vi "Simulation24Q1.vi"() -> ()   [LabVIEW 2024]
panel:
  out "out":dbl
  in  "in":dbl
  in  "function name":string
  in  "module path":path
  in  "Python path":path
  in  "Python version":string
  out "A2P":bool(c317)
  out "Actuator Valve 2":bool
  out "A1P":bool(c317)
  in  "Actuator Valve 1":bool
  out "Multi-Segment Pipe 5":bool(c317)
  out "A2_pipe":bool(c317)
  out "A1_pipe":bool(c317)
  out "Multi-Segment Pipe 10":bool(c317)
  out "Multi-Segment Pipe 9":bool(c317)
  in  "stop":bool
  in  "Oil Pump":bool
  out "S2":bool
  out "S1":bool
  out "Tank 2":dbl(slide) scale=0.0..100.0
  out "Multi-Segment Pipe 7":bool(c317)
  out "Multi-Segment Pipe 6":bool(c317)
  out "Multi-Segment Pipe 4":bool(c317)
  out "Multi-Segment Pipe 3":bool(c317)
  out "Multi-Segment Pipe 2":bool(c317)
  out "Tank 1":dbl(slide) scale=0.0..100.0
  # "Level Sensor"
  # "Oil Source"
  # "Level Sensor"
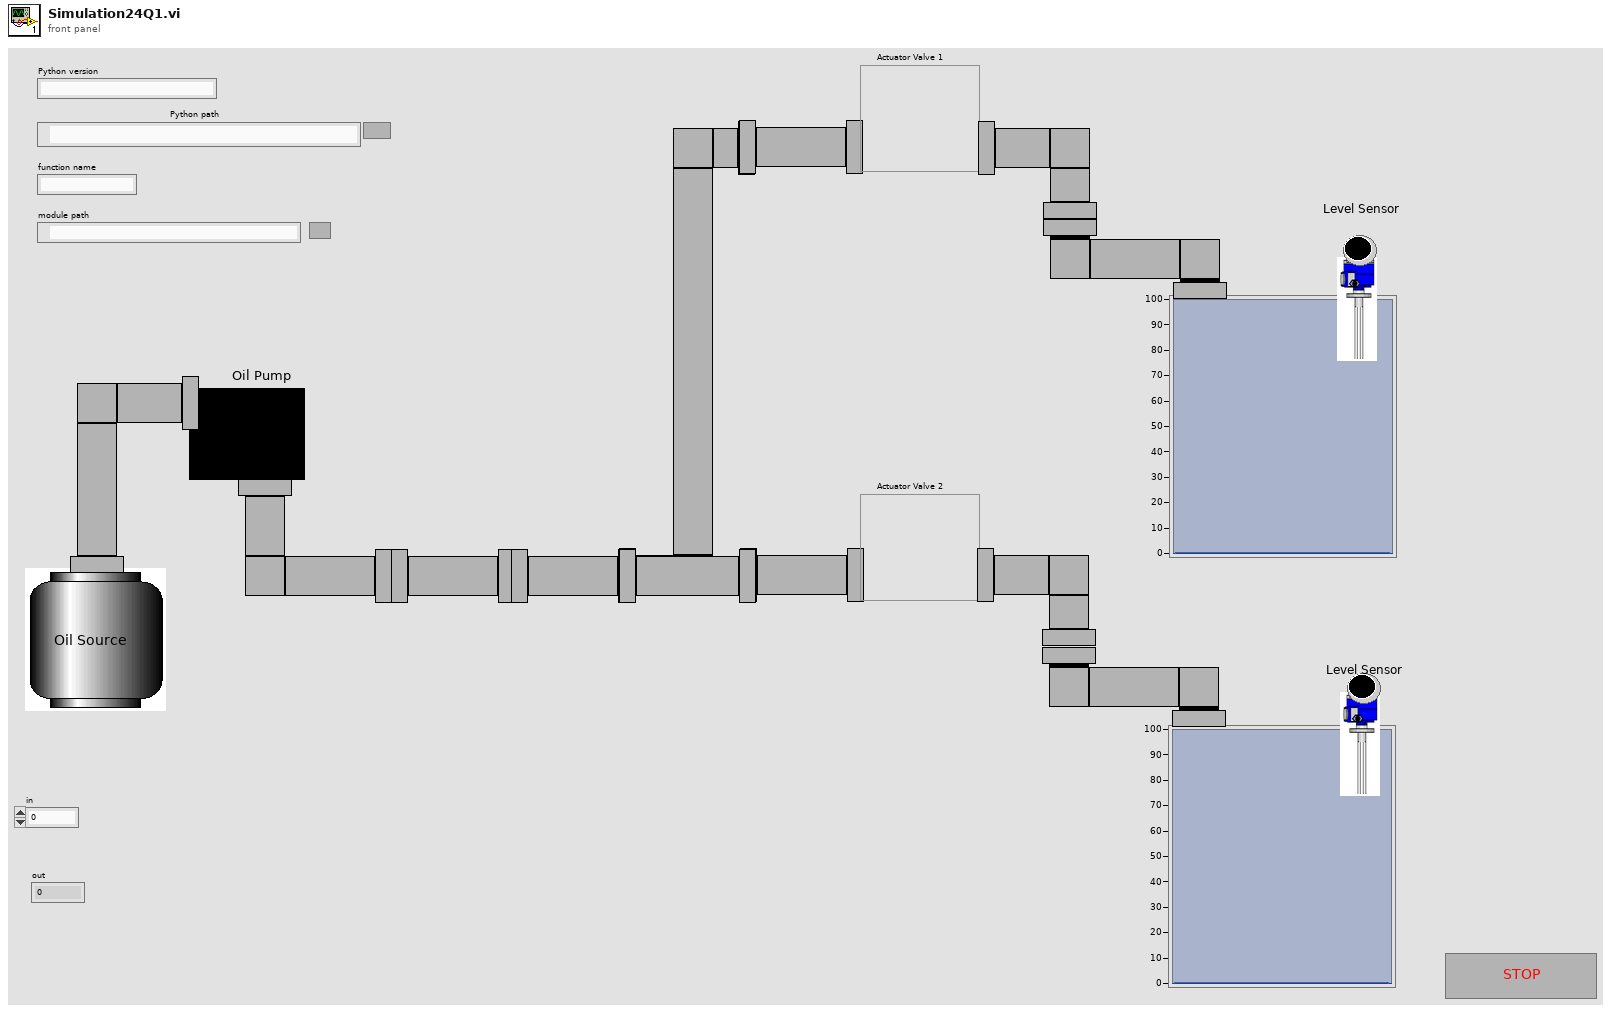
[diagram p1: front panel]
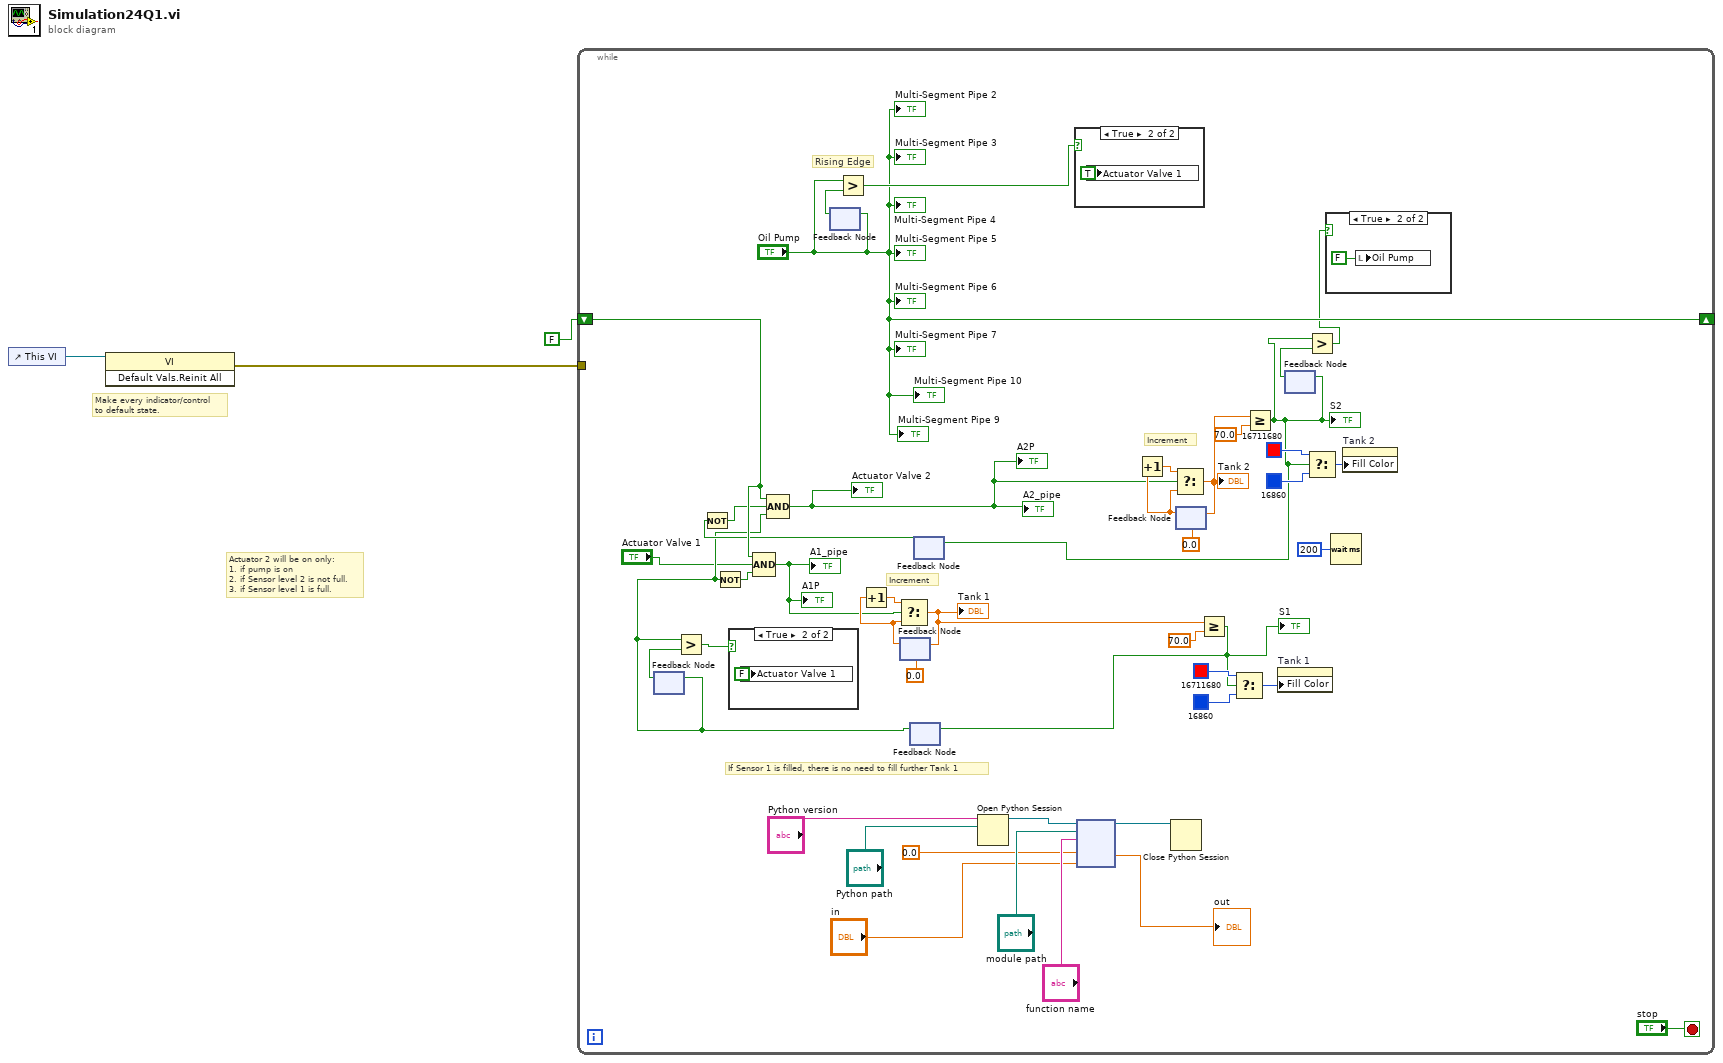
[diagram p0: block diagram]
diagram:
  # "Actuator 2 will be on only:\n1. if pump is on\n2. if Sensor level 2 is not full.\n3. if Sensor level 1 is full."
  # "Make every indicator/control\nto default state."
  n1 = control-ref of="This VI"() -> (w2:refnum<vi>)
  n2 = invoke class="VI" method="Default Vals.Reinit All"(reference=w2) -> (error out=w1:errorcluster)  [unwired: 2 in, 2 out]
  n3 = while {
    shift-right: ["Oil Pump"] -> _
    shift-left: FALSE -> [w46]
    tunnel: w1 -> [_]
    stop <- "stop" stop-if-true
    # "Increment"
    # "Increment"
    # "If Sensor 1 is filled, there is no need to fill further Tank 1"
    # "Rising Edge"
    n4 = feedback #1() -> (w28:bool)  [unwired: 1 in]
    n5 = feedback #2() -> (w22:bool)  [unwired: 1 in]
    n6 = feedback-in #2("Oil Pump") -> ()
    n7 = Greater?(x="Oil Pump", y=w22) -> (0:w21:bool)
    n8 = feedback #3(0.0) -> (w41:dbl)
    n9 = Increment(x=w41) -> (x+1=w40:dbl)
    n10 = feedback #4() -> (w23:bool)  [unwired: 1 in]
    n11 = feedback-in #1(w23) -> ()
    n12 = Greater?(x=w23, y=w28) -> (0:w27:bool)
    n13 = Not(x=w23) -> (.not. x?=w26:bool)
    n14 = case shown="True" w27 {
      frame False {
      }
      frame True {
        n15 = local write "Actuator Valve 1"(FALSE ("Actuator 1")) -> ()
      }
    }
    n16 = Compound Arithmetic op=AND(w46, "Actuator Valve 1", w26) -> (w16:bool)
    "A1_pipe" <- w16
    "A1P" <- w16
    n17 = Select(t=w40, s=w16, f=w41) -> (s? t:f=w7:dbl)
    "Tank 1" <- w7
    n18 = feedback-in #3(w7) -> ()
    n19 = feedback #5() -> (w25:bool)  [unwired: 1 in]
    n20 = Not(x=w25) -> (.not. x?=w24:bool)
    n21 = Compound Arithmetic op=AND(w46, w24, w23) -> (w14:bool)
    "A2_pipe" <- w14
    "Actuator Valve 2" <- w14
    "A2P" <- w14
    n22 = Open Python Session(python version="Python version", python path="Python path") -> (session out=w11:refnum<k35>)  [unwired: 1 in, 1 out]
    n23 = case shown="True" w21 {
      frame False {
      }
      frame True {
        n24 = local write "Actuator Valve 1"(TRUE ("Actuator 1")) -> ()
      }
    }
    n25 = node(w11, "module path", "function name", 0.0, "in") -> (w8:refnum<k35>, →"out":dbl)  [unwired: 2 in, 3 out]
    n26 = Close Python Session(session in=w8) -> ()  [unwired: 1 in, 1 out]
    n27 = feedback #6(0.0) -> (w42:dbl)
    n28 = Increment(x=w42) -> (x+1=w43:dbl)
    n29 = Select(t=w43, s=w14, f=w42) -> (s? t:f=w38:dbl)
    "Tank 2" <- w38
    n30 = feedback-in #6(w38) -> ()
    n31 = Greater Or Equal?(x=w7, y=70.0) -> (x >= y?=w29:bool)
    "S1" <- w29
    n32 = feedback-in #4(w29) -> ()
    n33 = Select(t=u32 16711680 ("Fill Color"), s=w29, f=u32 16860 ("Fill Color")) -> (s? t:f=w30:u32)
    n34 = Greater Or Equal?(x=w38, y=70.0) -> (x >= y?=w19:bool)
    "S2" <- w19
    n35 = feedback-in #5(w19) -> ()
    n36 = property on="Tank 1" class="Slide (strict)"("Fill Color"=w30) -> ()  [unwired: 2 in, 2 out]
    n37 = feedback #7() -> (w18:bool)  [unwired: 1 in]
    n38 = feedback-in #7(w19) -> ()
    n39 = Greater?(x=w19, y=w18) -> (0:w17:bool)
    n40 = Select(t=u32 16711680 ("Fill Color"), s=w19, f=u32 16860 ("Fill Color")) -> (s? t:f=w34:u32)
    n41 = case shown="True" w17 {
      frame False {
      }
      frame True {
        n42 = local write "Oil Pump"(FALSE ("Actuator 1")) -> ()
      }
    }
    n43 = Wait (ms)(milliseconds to wait=u32 200) -> ()  [unwired: 1 out]
    n44 = property on="Tank 2" class="Slide (strict)"("Fill Color"=w34) -> ()  [unwired: 2 in, 2 out]
    "Multi-Segment Pipe 2" <- "Oil Pump"
    "Multi-Segment Pipe 3" <- "Oil Pump"
    "Multi-Segment Pipe 4" <- "Oil Pump"
    "Multi-Segment Pipe 5" <- "Oil Pump"
    "Multi-Segment Pipe 6" <- "Oil Pump"
    "Multi-Segment Pipe 7" <- "Oil Pump"
    "Multi-Segment Pipe 9" <- "Oil Pump"
    "Multi-Segment Pipe 10" <- "Oil Pump"
  }
